vi "打开图片.vi"(1 "原图路径":path) -> (0 "模板":T1(plugin-control))   [LabVIEW 2014]
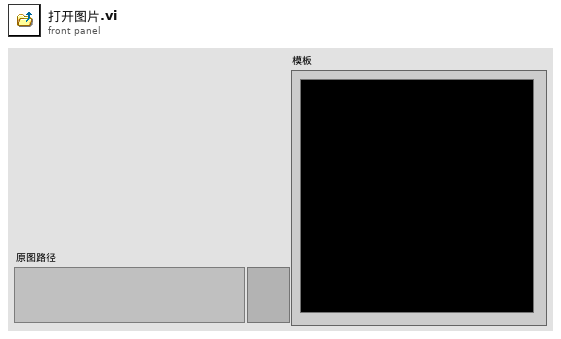
[diagram p1: front panel]
types:
  T1 = typedef "IMAQ Image.ctl" = refnum<image>
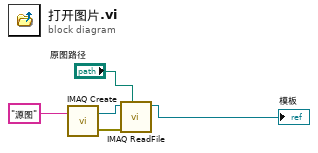
[diagram p0: block diagram]
diagram:
  n1 = call "IMAQ Create"("Image Name"="源图") -> ("New Image"=w4:T1, "error out"=w3:errorcluster)  [unwired: 3 in, 1 out]
  n2 = call "IMAQ ReadFile"("File Path"="原图路径", "error in (no error)"=w3, "Image"=w4) -> ("Image Out"=→"模板":T1)  [unwired: 2 in, 6 out]
